vi "Find All Embedded Data Logger Custom Devices.vi"(8 "error in":errorcluster, 11 "target in":refnum<k39>) -> (0 "error out":errorcluster, 2 "embedded data loggers":T1[](array[typedef]) format="%.0x", 3 "target out":refnum<k39>)   [LabVIEW 2027, in "Embedded Data Logger Scripting.lvlib"]
uses:
  Embedded Data Logger Scripting.lvlib
  C:/NetCore/niveristand-embedded-data-logger-custom-device/Source/Scripting/Custom Device/Find All Embedded Data Logger Custom Devices.vi/NationalInstruments.VeriStand.SystemDefinitionAPI
  NationalInstruments.VeriStand.SystemDefinitionAPI
  Shared/Constants.vi
  Shared/Embedded Data Logger Shared.lvlib
  C:/NetCoreDLL/NationalInstruments.VeriStand.SystemDefinitionAPI.dll
  NetCoreDLL/NationalInstruments.VeriStand.SystemDefinitionAPI.dll
  <vilib>/NI VeriStand/Custom Device API/Custom Device Item Ref.ctl
  <vilib>/NI VeriStand/Custom Device API/Custom Device API.lvlib
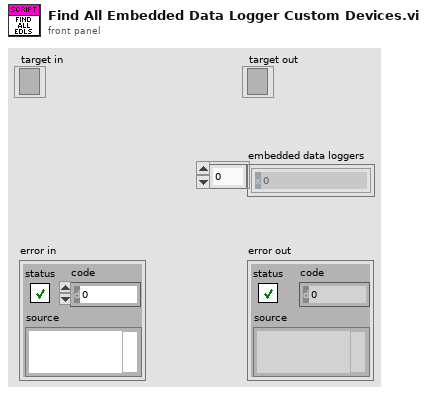
[diagram p1: front panel]
types:
  T1 = typedef "Custom Device API.lvlib/Custom Device Item Ref.ctl" = u64
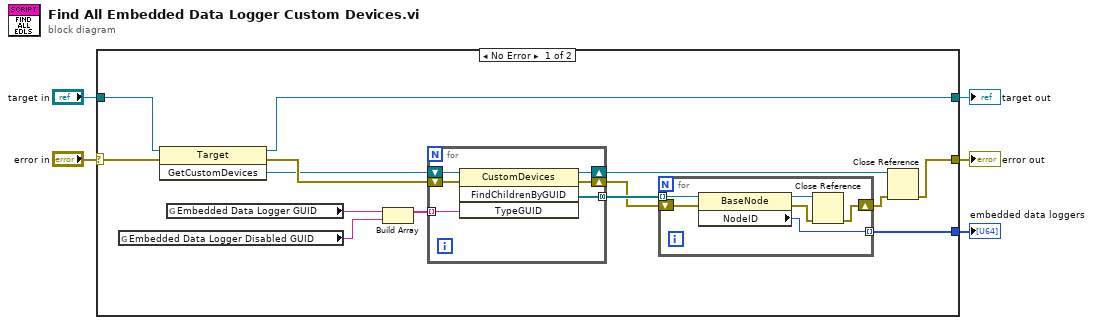
[diagram p0: block diagram]
diagram:
  n1 = case shown="No Error" "error in" {
    selector: "error in" -> [w16 w32]
    tunnel: "target in" -> [w17 w33]
    tunnel: [w11 w33] -> w3
    tunnel: [w8 w32] -> w2
    tunnel: [w12 _] -> w1
    frame No Error {
      n2 = global read "Constants.vi" "Embedded Data Logger Disabled GUID"() -> (w6:string)
      n3 = invoke class="Target" method="GetCustomDevices"(reference=w17, error in=w16) -> (reference out=w11:refnum<k39>, error out=w19:errorcluster, "GetCustomDevices"=w18:refnum<k39>)  [unwired: 1 in]
      n4 = global read "Constants.vi" "Embedded Data Logger GUID"() -> (w15:string)
      n5 = Build Array(w15, w6) -> (w7:string[])
      n6 = for {
        tunnel: w7 -> [w23] mode=indexing
        tunnel: [w22] -> w14 mode=concatenating
        shift-right: [w21] -> w13
        shift-left: w19 -> [w25]
        shift-right: [w20] -> w9
        shift-left: w18 -> [w24]
        n7 = invoke class="CustomDevices" method="FindChildrenByGUID"(reference=w24, error in=w25, "TypeGUID"=w23) -> (reference out=w20:refnum<k39>, error out=w21:errorcluster, "FindChildrenByGUID"=w22:refnum<k39>[])  [unwired: 1 in, 1 out]
      }
      n8 = for {
        tunnel: w14 -> [w31] mode=indexing
        tunnel: [w27] -> w12 mode=indexing
        shift-right: [w26] -> w10
        shift-left: w13 -> [w30]
        n9 = property class="BaseNode"(reference=w31, error in=w30) -> (reference out=w29:refnum<k39>, error out=w28:errorcluster, "NodeID"=w27:u64)
        n10 = Close Reference(reference=w29, error in (no error)=w28) -> (error out=w26:errorcluster)
      }
      n11 = Close Reference(reference=w9, error in (no error)=w10) -> (error out=w8:errorcluster)
    }
    frame Error {
    }
  }
  "target out" <- w3
  "error out" <- w2
  "embedded data loggers" <- w1
